vi "Polymorphic - Asynchronous Write.vi"   [LabVIEW 2021]
doc: "Send an asychronous message to the DAQiFi device."
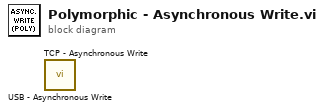
[diagram p0: block diagram]
diagram:
  n1 = call "USB - Asynchronous Write.vi"() -> ()  [unwired: 10 in, 2 out]
  n2 = call "TCP - Asynchronous Write.vi"() -> ()  [unwired: 10 in, 2 out]
